vi "Is VI Server Required.vi"(8 "error in (no error)":errorcluster, 11 "Numeric Assertion in":refnum<class "Numeric Assertion.lvclass">) -> (0 "error out":errorcluster, 2 "VI Server Required?":bool, 3 "Numeric Assertion out":refnum<class "Numeric Assertion.lvclass">)   [LabVIEW 2020, in "MacroAssert.lvlib" / "Numeric Assertion.lvclass"]
doc: "Outputs whether VI Server is required to perform the given step."
uses:
  Numeric Assertion.lvclass
  Numeric Assertion.lvclass/Numeric Assertion.ctl
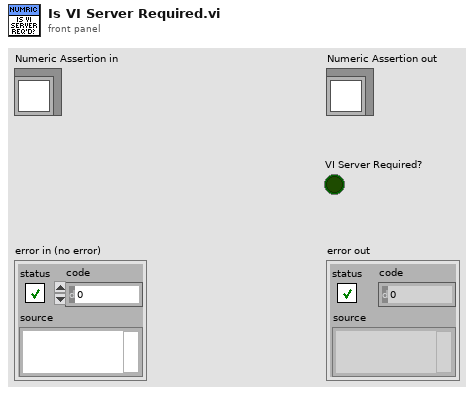
[diagram p1: front panel]
types:
  T1 = typedef "MacroAssert.lvlib/Numeric Assertion.lvclass/Numeric Assertion Type.ctl" = enum16{"Numeric Ctl Value", "Array Ctl Size", "Ctl Width Property", "Ctl Height Property", "VI Width", "VI Height", "Window Width", "Window Height", "Window Scale", "Number of Displays", "Highest Display Scale"}
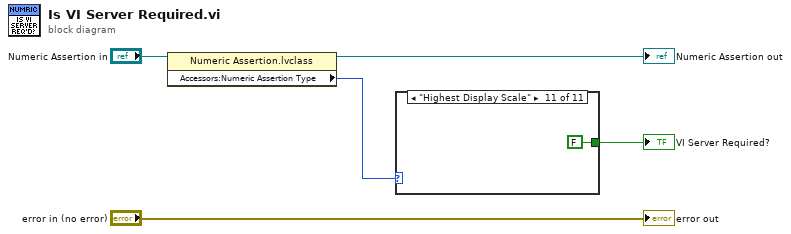
[diagram p0: block diagram]
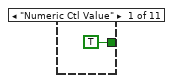
[diagram p2: hidden frame]
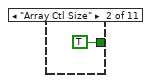
[diagram p3: hidden frame]
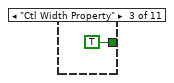
[diagram p4: hidden frame]
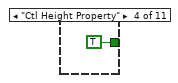
[diagram p5: hidden frame]
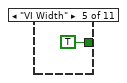
[diagram p6: hidden frame]
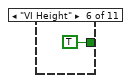
[diagram p7: hidden frame]
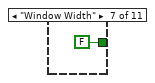
[diagram p8: hidden frame]
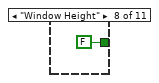
[diagram p9: hidden frame]
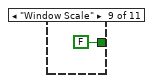
[diagram p10: hidden frame]
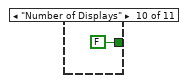
[diagram p11: hidden frame]
diagram:
  n1 = property class="Numeric Assertion.lvclass"(reference="Numeric Assertion in") -> (reference out=→"Numeric Assertion out":refnum<class "Numeric Assertion.lvclass">, "Accessors:Numeric Assertion Type"=w1:T1)  [unwired: 1 in, 1 out]
  n2 = case shown="\"Highest Display Scale\"" w1 {
    tunnel: [TRUE TRUE TRUE TRUE TRUE TRUE FALSE FALSE FALSE FALSE FALSE] -> w2
    frame "Numeric Ctl Value" {
    }
    frame "Array Ctl Size" {
    }
    frame "Ctl Width Property" {
    }
    frame "Ctl Height Property" {
    }
    frame "VI Width" {
    }
    frame "VI Height" {
    }
    frame "Window Width" {
    }
    frame "Window Height" {
    }
    frame "Window Scale" {
    }
    frame "Number of Displays" {
    }
    frame "Highest Display Scale" {
    }
  }
  "VI Server Required?" <- w2
  "error out" <- "error in (no error)"
